vi "niRFUtil MASMT Util Resample_Create Prototype Filter (SGL).vi"(8 "error in (no error)":errorcluster, 10 "anti-aliasing?":bool=TRUE, 11 "FIR filter specifications":T1={"alias rejection (dB)"=120.0, "normalized bandwidth"=0.4536}) -> (0 "error out":errorcluster, 2 "decimation factor":i32, 3 "Coefficients":sgl[](array[numeric]))   [LabVIEW 2015, in "niRFUtil.lvlib"]
uses:
  niRFUtil.lvlib
  <vilib>/Analysis/NI_AALPro.lvlib
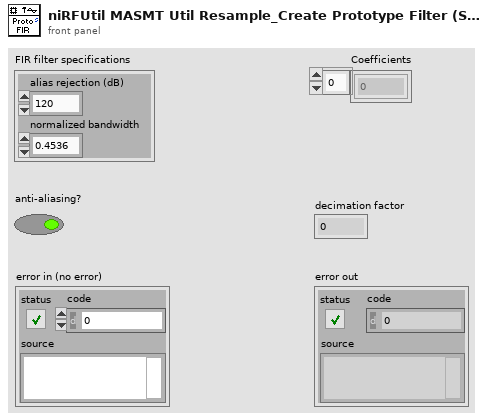
[diagram p1: front panel]
types:
  T1 = cluster{"alias rejection (dB)":sgl, "normalized bandwidth":sgl}
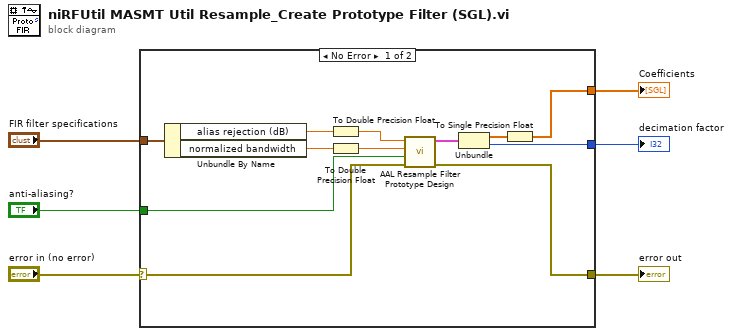
[diagram p0: block diagram]
diagram:
  n1 = case shown="No Error" "error in (no error)" {
    selector: "error in (no error)" -> [w13 w19]
    tunnel: [w7 _] -> w6
    tunnel: [w16 _] -> w5
    tunnel: "anti-aliasing?" -> [w15 _]
    tunnel: [w14 w19] -> w3
    tunnel: "FIR filter specifications" -> [w10 _]
    frame No Error {
      n2 = Unbundle By Name(w10) -> ("alias rejection (dB)"=w12:sgl, "normalized bandwidth"=w11:sgl)
      n3 = To Double Precision Float(number=w12) -> (double precision float=w9:dbl)
      n4 = To Double Precision Float(number=w11) -> (double precision float=w8:dbl)
      n5 = call <vilib>:"AAL Resample Filter Prototype Design.vi"("error in (no error)"=w13, "alias free"=w15, "normalized bandwidth"=w8, "A stop [dB]"=w9) -> ("error out"=w14:errorcluster, "filter prototype"=w18:cluster{"coefficients":dbl[], "factor":i32})  [unwired: 5 in, 1 out]
      n6 = Unbundle(w18) -> ("coefficients"=w17:dbl[], "factor"=w16:i32)
      n7 = To Single Precision Float(number=w17) -> (single precision float=w7:sgl[])
    }
    frame Error {
    }
  }
  "decimation factor" <- w5
  "Coefficients" <- w6
  "error out" <- w3
